vi "keysight_write.vi"(0 "error in":errorcluster, 2 "command":string, 3 "Connection":T1={"Type"=0, "VISA"="TCPIP0::192.168.0.8::inst0::INSTR", "GPIB"="10"} {"Type" items=["VISA", "GPIB"]}) -> (1 "error out":errorcluster)   [LabVIEW 2013]
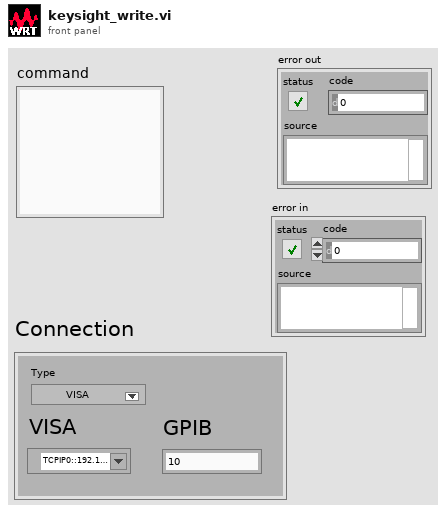
[diagram p1: front panel]
types:
  T1 = cluster{"Type":u16, "VISA":refnum<visa-resource-name>, "GPIB":string}
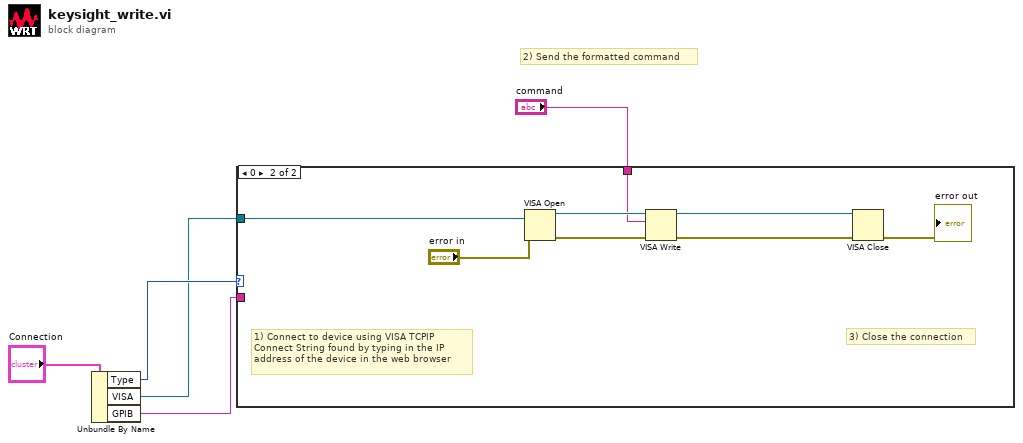
[diagram p0: block diagram]
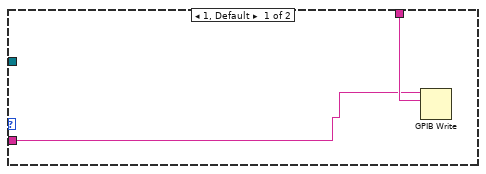
[diagram p2: hidden frame]
diagram:
  # "2) Send the formatted command"
  n1 = Unbundle By Name("Connection") -> ("Type"=w3:u16, "VISA"=w2:refnum<visa-resource-name>, "GPIB"=w1:string)
  n2 = case shown="0" w3 {
    tunnel: "command" -> [w7 w10]
    tunnel: w1 -> [w6 _]
    tunnel: w2 -> [_ w8]
    frame 1, Default {
      n3 = GPIB Write(0:w6, 1:w7) -> ()  [unwired: 3 in, 2 out]
    }
    frame 0 {
      # "3) Close the connection"
      # "1) Connect to device using VISA TCPIP Connect String found by typing in the IP address of the device in the web browser"
      n4 = VISA Open(error in (no error)="error in", VISA resource name=w8) -> (VISA resource name=w11:refnum<visa-resource-name>, error out=w12:errorcluster)  [unwired: 3 in]
      n5 = VISA Write(VISA resource name=w11, write buffer=w10, error in (no error)=w12) -> (VISA resource name out=w13:refnum<visa-resource-name>, error out=w14:errorcluster)  [unwired: 1 out]
      n6 = VISA Close(VISA resource name=w13, error in (no error)=w14) -> (error out=→"error out":errorcluster)
    }
  }
